vi "ConstructorTypeString.vi"(5 "list":string, 9 "terminals":refnum<class "Terminal.lvclass">[](array[class])) -> (4 "constructor string":string)   [LabVIEW 2014, in "Raspberry Pi Compatible Compiler for LabVIEW.lvlib" / "Function.lvclass"]
uses:
  Function.lvclass
  Terminal/Terminal.lvclass
  Python/Parsing/Python Functions.lvlib
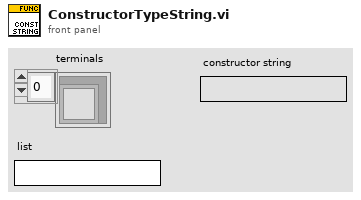
[diagram p1: front panel]
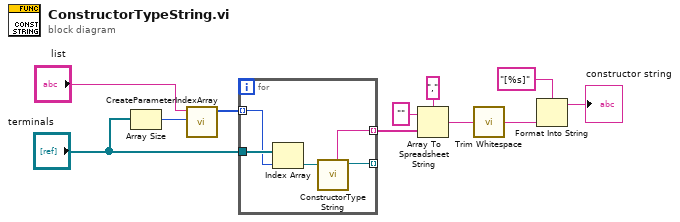
[diagram p0: block diagram]
diagram:
  n1 = Array Size(array="terminals") -> (size(s)=w10:i32)
  n2 = call "CreateParameterIndexArray.vi"("length"=w10, "list"="list") -> ("Array"=w9:i32[])  [unwired: 9 in]
  n3 = for {
    tunnel: w9 -> [w15] mode=indexing
    tunnel: "terminals" -> [w16]
    tunnel: [w13] -> _ mode=indexing
    tunnel: [w12] -> w7 mode=indexing
    n4 = Index Array(array=w16, index=w15) -> (element=w14:refnum<class "Terminal.lvclass">)
    n5 = call "ConstructorTypeString.vi"("Terminal in"=w14) -> ("Terminal out"=w13:refnum<class "Terminal.lvclass">, "constructor string"=w12:string)  [unwired: 6 in, 1 out]
  }
  n6 = Array To Spreadsheet String(delimiter (Tab)=",", array=w7, 3:"" ("format string")) -> (spreadsheet string=w4:string)
  n7 = call <vilib>:"Trim Whitespace.vi"("string"=w4) -> ("trimmed string"=w3:string)  [unwired: 1 in]
  n8 = Format Into String(format string="[%s]", w3) -> (resulting string=→"constructor string":string)  [unwired: 2 in, 1 out]
